vi "Apodization.vi"(6 "STEPS":i32, 9 "POSITION":i32, 10 "y":dbl[](array[numeric]), 11 "x":dbl[](array[numeric])) -> (3 "Apodized_y":dbl[](array[numeric]))   [LabVIEW 2019]
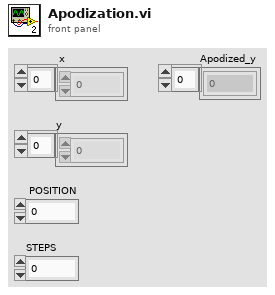
[diagram p1: front panel]
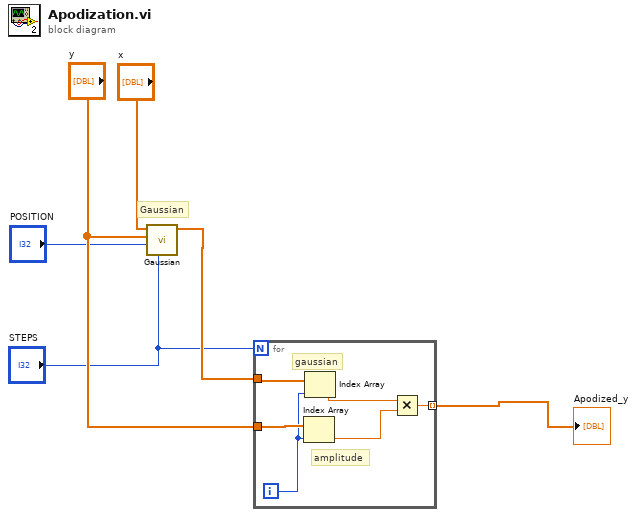
[diagram p0: block diagram]
diagram:
  # "Gaussian"
  n1 = call "Gaussian.vi"("STEPS"="STEPS", "POSITION"="POSITION", "y"="y", "x"="x") -> ("Gaussian"=w4:dbl[])  [unwired: 7 in]
  n2 = for {
    N: "STEPS" -> [_]
    tunnel: w4 -> [w12]
    tunnel: "y" -> [w11]
    tunnel: [w7] -> w6 mode=indexing
    i -> [w10]
    # "amplitude"
    # "gaussian"
    n3 = Index Array(array=w11, index=w10) -> (element=w8:dbl)
    n4 = Index Array(array=w12, index=w10) -> (element=w9:dbl)
    n5 = Multiply(x=w9, y=w8) -> (x*y=w7:dbl)
  }
  "Apodized_y" <- w6
